vi "Disconnect TypeDef.vi"(1 "Variant":variant) -> (0 "Variant Out":variant)   [LabVIEW 2013, in "Caraya.lvlib" / "Assert.lvclass"]
uses:
  classes/Assert/Assert.lvclass
  <vilib>/Utility/VariantDataType/VariantType.lvlib
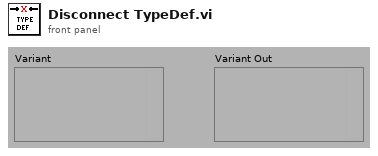
[diagram p1: front panel]
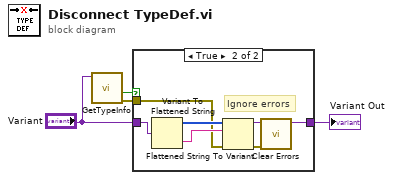
[diagram p0: block diagram]
diagram:
  n1 = call <vilib>:"GetTypeInfo.vi"("Variant"="Variant") -> ("error out"=w1:errorcluster, "HasTypedef"=w2:bool)  [unwired: 6 in, 3 out]
  n2 = case shown="True" w2 {
    tunnel: [w5 w10] -> w4
    tunnel: "Variant" -> [w5 w7]
    tunnel: w1 -> [_ w6]
    frame False {
    }
    frame True {
      # "Ignore errors"
      n3 = Variant To Flattened String(Variant=w7) -> (data string=w8:string, 1:w9:i16[])
      n4 = Flattened String To Variant(4:w6, 6:w8, 7:w9) -> (0:w11:errorcluster, 3:w10:variant)
      n5 = call <vilib>:"Clear Errors.vi"("error in (no error)"=w11) -> ()  [unwired: 6 in, 1 out]
    }
  }
  "Variant Out" <- w4
